vi "Add Verbose Explanation.vi"(7 "overwrite?":bool=TRUE, 9 "error in (no error)":errorcluster, 10 "Verbose Explanation":string, 11 "Properties":refnum<class "Properties.lvclass">) -> (1 "error out":errorcluster, 3 "Properties":refnum<class "Properties.lvclass">)   [LabVIEW 2020, in "Caraya.lvlib" / "Properties.lvclass"]
uses:
  Properties.lvclass
  Properties.lvclass/Properties.ctl
  Test Manager Message Verbose/TestManagerMsg.Verbose.lvclass
  Caraya.lvlib
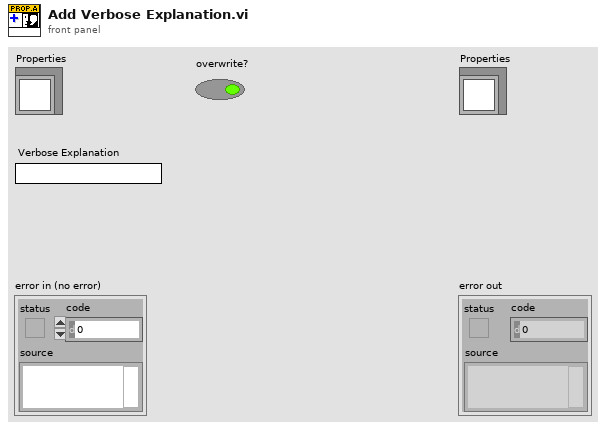
[diagram p1: front panel]
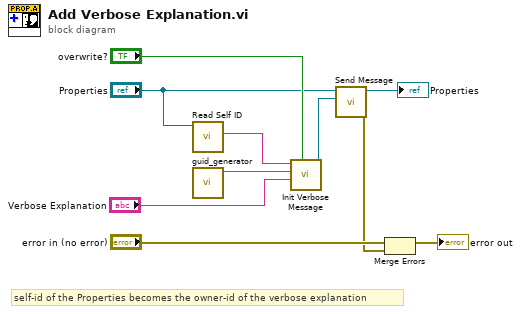
[diagram p0: block diagram]
diagram:
  # "self-id of the Properties becomes the owner-id of the verbose explanation"
  n1 = call "Read Self ID.vi"("Properties in"="Properties") -> ("self-id"=w2:string)  [unwired: 9 in, 1 out]
  n2 = call "guid_generator.vi"() -> ("guid"=w1:string)  [unwired: 11 in]
  n3 = call "Init Verbose Message.vi"("overwrite?"="overwrite?", "explanation"="Verbose Explanation", "self-id"=w1, "owner-id"=w2) -> ("Message"=w5:refnum<class "TestManagerMsg.lvclass">)  [unwired: 7 in]
  n4 = call "Send Message.vi"("TestManagerMsg"=w5, "Properties in"="Properties") -> ("error out"=w4:errorcluster, "Properties out"=→"Properties":refnum<class "Properties.lvclass">)  [unwired: 8 in]
  n5 = Merge Errors("error in (no error)", w4) -> (→"error out":errorcluster)
